vi "Read Roles.vi"(8 "error in (no error)":errorcluster, 11 "PrepareTriplePassPlay in":refnum<class "PrepareTriplePassPlay.lvclass">) -> (0 "error out":errorcluster, 2 "Roles":T1, 3 "PrepareTriplePassPlay out":refnum<class "PrepareTriplePassPlay.lvclass">)   [LabVIEW 2023, in "PrepareTriplePassPlay.lvclass"]
uses:
  PrepareTriplePassPlay.lvclass
  PreparePassReceiverRole_class/PreparePassReceiverRole.lvclass
  AttackerStopRole_class/AttackerStopRole.lvclass
  PrepareTriplePassPlay.lvclass/PrepareTriplePassPlay.ctl
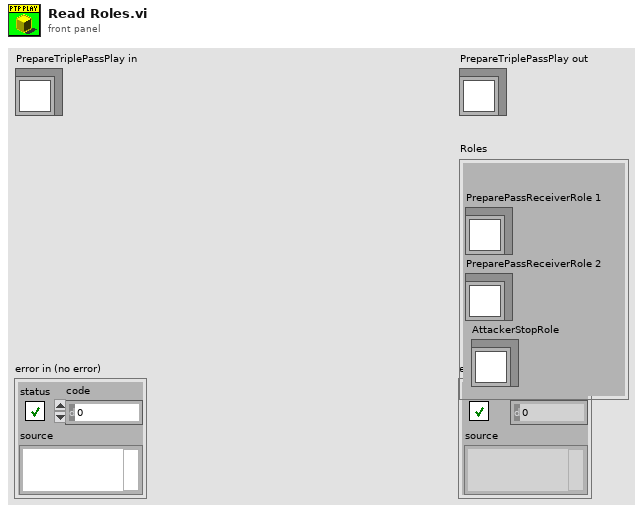
[diagram p1: front panel]
types:
  T1 = cluster{"PreparePassReceiverRole 1":refnum<class "PreparePassReceiverRole.lvclass">, "PreparePassReceiverRole 2":refnum<class "PreparePassReceiverRole.lvclass">, "AttackerStopRole":refnum<class "AttackerStopRole.lvclass">}
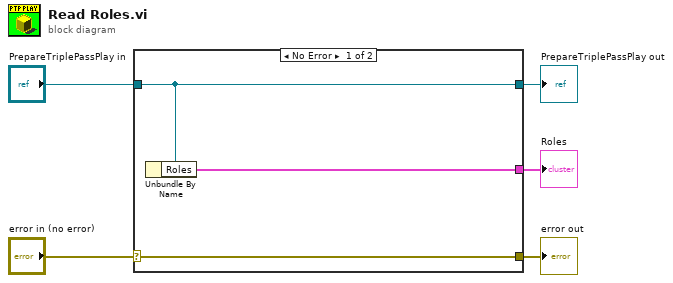
[diagram p0: block diagram]
diagram:
  n1 = case shown="No Error" "error in (no error)" {
    selector: "error in (no error)" -> [w8 w9]
    tunnel: [w8 w9] -> w4
    tunnel: [w7 w10] -> w2
    tunnel: "PrepareTriplePassPlay in" -> [w7 w10]
    tunnel: [w6 _] -> w1
    frame No Error {
      n2 = Unbundle By Name(w7) -> ("Roles"=w6:T1)
    }
    frame Error {
    }
  }
  "error out" <- w4
  "PrepareTriplePassPlay out" <- w2
  "Roles" <- w1
